vi "RxTx.vi"(8 "error in (no error)":errorcluster) -> (0 "error out":errorcluster)   [LabVIEW 2018]
uses:
  RxTx/RxTx.lvclass
  RxTx/RxTx.lvclass/RxTx.ctl
  <vilib>/addons/_JKI Toolkits/Caraya/classes/Assert/Assert Equal Value_Variant.vi
  <vilib>/addons/_JKI Toolkits/Caraya/classes/Assert/Assert Error.vi
  <vilib>/addons/_JKI Toolkits/Caraya/classes/Test/Test.lvclass
  <vilib>/addons/_JKI Toolkits/Caraya/classes/Assert/Assert.lvclass
panel:
  in  "RxTx in 2":refnum<class "RxTx.lvclass">
  in  "RxTx in":refnum<class "RxTx.lvclass">
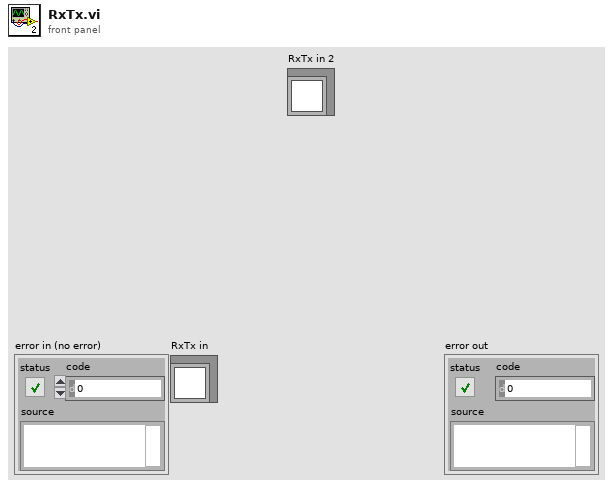
[diagram p1: front panel]
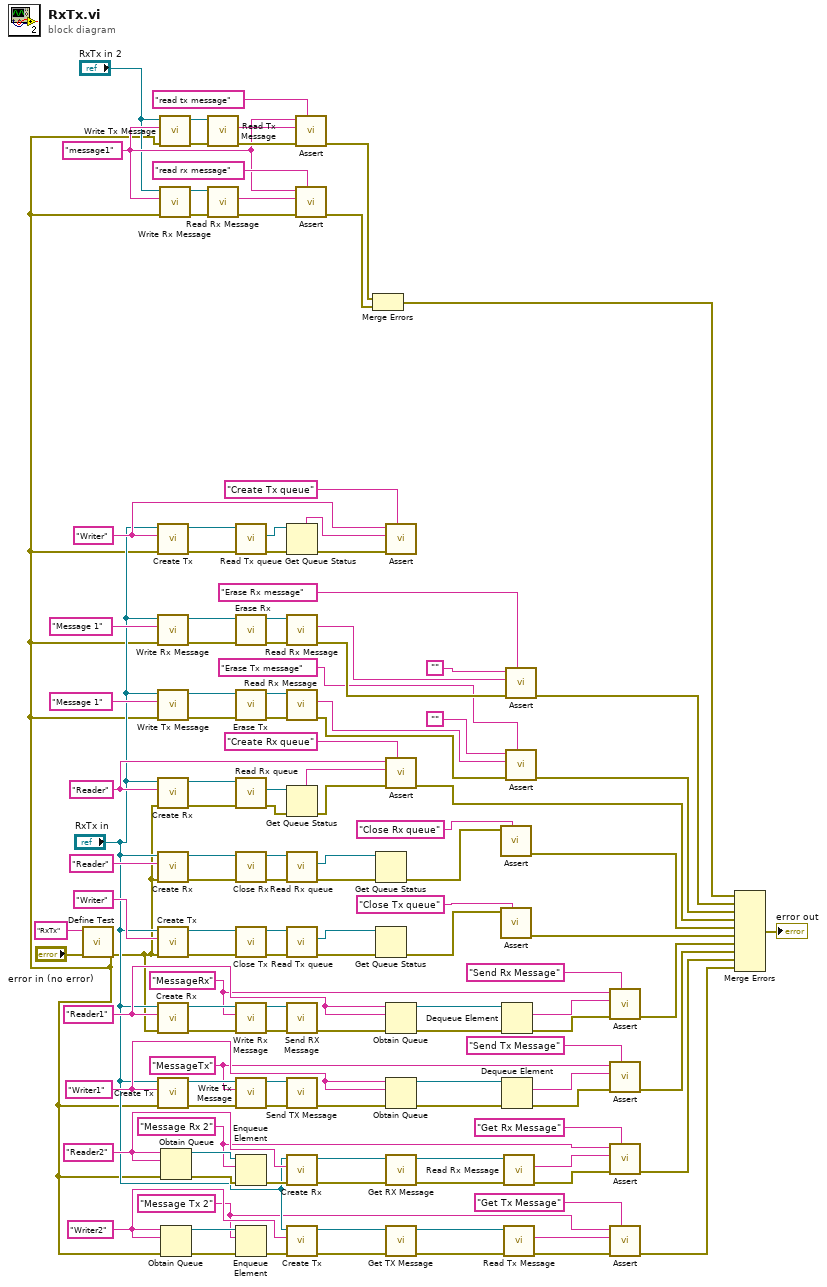
[diagram p0: block diagram]
diagram:
  w4 = "message1" ("Label (VI Title)")
  w18 = "Message Tx 2" ("Rx Message")
  w26 = "Writer2" ("Rx Message")
  w33 = "Message Rx 2" ("Rx Message")
  w40 = "Reader2" ("Rx Message")
  w46 = "MessageTx" ("Rx Message")
  w48 = "Writer1" ("Rx Message")
  w60 = "MessageRx" ("Rx Message")
  w64 = "Reader1" ("Rx Message")
  w97 = "Writer" ("Rx Message")
  w100 = "Reader" ("Rx Message")
  n1 = call <vilib>:"Define Test.vi"("error in (no error)"="error in (no error)", "Label (VI Title)"="RxTx") -> ("error out"=w2:errorcluster)  [unwired: 8 in, 1 out]
  n2 = call "Create Tx.vi"("error in (no error)"=w2, "Writer Name"=w97, "RxTx in"="RxTx in") -> ("error out"=w91:errorcluster, "RxTx out"=w92:refnum<class "RxTx.lvclass">)  [unwired: 7 in]
  n3 = call "Write Rx Message.vi"("error in (no error)"=w2, "Rx Message"="Message 1", "RxTx in"="RxTx in") -> ("error out"=w126:errorcluster, "RxTx out"=w125:refnum<class "RxTx.lvclass">)  [unwired: 7 in]
  n4 = call "Write Tx Message.vi"("error in (no error)"=w2, "Tx Message"="Message 1" ("Rx Message"), "RxTx in"="RxTx in") -> ("error out"=w112:errorcluster, "RxTx out"=w111:refnum<class "RxTx.lvclass">)  [unwired: 7 in]
  n5 = call "Create Rx.vi"("error in (no error)"=w2, "Reader Name"=w100, "RxTx in"="RxTx in") -> ("error out"=w106:errorcluster, "RxTx out"=w105:refnum<class "RxTx.lvclass">)  [unwired: 7 in]
  n6 = call "Create Rx.vi"("error in (no error)"=w2, "Reader Name"="Reader" ("Rx Message"), "RxTx in"="RxTx in") -> ("error out"=w88:errorcluster, "RxTx out"=w87:refnum<class "RxTx.lvclass">)  [unwired: 7 in]
  n7 = call "Create Tx.vi"("error in (no error)"=w2, "Writer Name"="Writer" ("Rx Message"), "RxTx in"="RxTx in") -> ("error out"=w79:errorcluster, "RxTx out"=w78:refnum<class "RxTx.lvclass">)  [unwired: 7 in]
  n8 = call "Create Rx.vi"("error in (no error)"=w2, "Reader Name"=w64, "RxTx in"="RxTx in") -> ("error out"=w69:errorcluster, "RxTx out"=w66:refnum<class "RxTx.lvclass">)  [unwired: 7 in]
  n9 = call "Create Tx.vi"("error in (no error)"=w2, "Writer Name"=w48, "RxTx in"="RxTx in") -> ("error out"=w56:errorcluster, "RxTx out"=w55:refnum<class "RxTx.lvclass">)  [unwired: 7 in]
  n10 = call "Write Tx Message.vi"("error in (no error)"=w2, "Tx Message"=w4, "RxTx in"="RxTx in 2") -> ("error out"=w15:errorcluster, "RxTx out"=w8:refnum<class "RxTx.lvclass">)  [unwired: 7 in]
  n11 = call "Write Rx Message.vi"("error in (no error)"=w2, "Rx Message"=w4, "RxTx in"="RxTx in 2") -> ("error out"=w13:errorcluster, "RxTx out"=w7:refnum<class "RxTx.lvclass">)  [unwired: 7 in]
  n12 = Obtain Queue(name (unnamed)=w40, element data type=w40, error in (no error)=w2) -> (queue out=w42:refnum<queue>, error out=w43:errorcluster)  [unwired: 2 in, 1 out]
  n13 = Obtain Queue(name (unnamed)=w26, element data type=w26, error in (no error)=w2) -> (queue out=w30:refnum<queue>, error out=w29:errorcluster)  [unwired: 2 in, 1 out]
  n14 = call "Read Tx Message.vi"("error in (no error)"=w15, "RxTx in"=w8) -> ("error out"=w14:errorcluster, "Tx Message"=w5:string)  [unwired: 7 in, 1 out]
  n15 = call "Read Rx Message.vi"("error in (no error)"=w13, "RxTx in"=w7) -> ("error out"=w12:errorcluster, "Rx Message"=w6:string)  [unwired: 7 in, 1 out]
  n16 = call "Read Tx queue.vi"("error in (no error)"=w91, "RxTx in"=w92) -> ("error out"=w94:errorcluster, "Tx"=w93:refnum<queue>)  [unwired: 7 in, 1 out]
  n17 = call "Erase Rx.vi"("error in (no error)"=w126, "RxTx in"=w125) -> ("error out"=w124:errorcluster, "RxTx out"=w119:refnum<class "RxTx.lvclass">)  [unwired: 8 in]
  n18 = call "Erase Tx.vi"("error in (no error)"=w112, "RxTx in"=w111) -> ("error out"=w109:errorcluster, "RxTx out"=w110:refnum<class "RxTx.lvclass">)  [unwired: 8 in]
  n19 = call "Read Rx queue.vi"("error in (no error)"=w106, "RxTx in"=w105) -> ("error out"=w103:errorcluster, "Rx"=w104:refnum<queue>)  [unwired: 7 in, 1 out]
  n20 = call "Close Rx.vi"("error in (no error)"=w88, "RxTx in"=w87) -> ("error out"=w86:errorcluster, "RxTx out"=w85:refnum<class "RxTx.lvclass">)  [unwired: 8 in]
  n21 = call "Close Tx.vi"("error in (no error)"=w79, "RxTx in"=w78) -> ("error out"=w76:errorcluster, "RxTx out"=w75:refnum<class "RxTx.lvclass">)  [unwired: 8 in]
  n22 = call "Write Rx Message.vi"("error in (no error)"=w69, "Rx Message"=w60, "RxTx in"=w66) -> ("error out"=w68:errorcluster, "RxTx out"=w67:refnum<class "RxTx.lvclass">)  [unwired: 7 in]
  n23 = call "Write Tx Message.vi"("error in (no error)"=w56, "Tx Message"=w46, "RxTx in"=w55) -> ("error out"=w54:errorcluster, "RxTx out"=w53:refnum<class "RxTx.lvclass">)  [unwired: 7 in]
  n24 = Enqueue Element(queue=w42, element=w33, error in (no error)=w43) -> (error out=w41:errorcluster)  [unwired: 1 in, 2 out]
  n25 = Enqueue Element(queue=w30, element=w18, error in (no error)=w29) -> (error out=w28:errorcluster)  [unwired: 1 in, 2 out]
  n26 = Get Queue Status(queue=w93, error in (no error)=w94) -> (queue name=w96:string, error out=w95:errorcluster)  [unwired: 1 in, 6 out]
  n27 = call "Read Rx Message.vi"("error in (no error)"=w124, "RxTx in"=w119) -> ("error out"=w123:errorcluster, "Rx Message"=w122:string)  [unwired: 7 in, 1 out]
  n28 = call "Read Rx Message.vi"("error in (no error)"=w109, "RxTx in"=w110) -> ("error out"=w113:errorcluster, "Rx Message"=w114:string)  [unwired: 7 in, 1 out]
  n29 = Get Queue Status(queue=w104, error in (no error)=w103) -> (queue name=w101:string, error out=w102:errorcluster)  [unwired: 1 in, 6 out]
  n30 = call "Read Rx queue.vi"("error in (no error)"=w86, "RxTx in"=w85) -> ("error out"=w82:errorcluster, "Rx"=w84:refnum<queue>)  [unwired: 7 in, 1 out]
  n31 = call "Read Tx queue.vi"("error in (no error)"=w76, "RxTx in"=w75) -> ("error out"=w73:errorcluster, "Tx"=w74:refnum<queue>)  [unwired: 7 in, 1 out]
  n32 = call "Send RX Message.vi"("error in (no error)"=w68, "RxTx in"=w67) -> ("error out"=w65:errorcluster)  [unwired: 8 in, 1 out]
  n33 = call "Send TX Message.vi"("error in (no error)"=w54, "RxTx in"=w53) -> ("error out"=w52:errorcluster)  [unwired: 8 in, 1 out]
  n34 = call "Create Rx.vi"("error in (no error)"=w41, "Reader Name"=w40, "RxTx in"="RxTx in") -> ("error out"=w39:errorcluster, "RxTx out"=w38:refnum<class "RxTx.lvclass">)  [unwired: 7 in]
  n35 = call "Create Tx.vi"("error in (no error)"=w28, "Writer Name"=w26, "RxTx in"="RxTx in") -> ("error out"=w24:errorcluster, "RxTx out"=w25:refnum<class "RxTx.lvclass">)  [unwired: 7 in]
  n36 = call-poly <vilib>:"Assert.vi"("Label"="read tx message" ("Label (VI Title)"), "error in (no error)"=w14, "Actual"=w5, "Expected"=w4) -> ("error out"=w16:errorcluster)  [unwired: 6 in, 1 out]
  n37 = call-poly <vilib>:"Assert.vi"("Label"="read rx message" ("Label (VI Title)"), "error in (no error)"=w12, "Actual"=w6, "Expected"=w4) -> ("error out"=w11:errorcluster)  [unwired: 6 in, 1 out]
  n38 = Merge Errors(w16, w11) -> (w1:errorcluster)
  n39 = Get Queue Status(queue=w84, error in (no error)=w82) -> (error out=w83:errorcluster)  [unwired: 1 in, 7 out]
  n40 = Get Queue Status(queue=w74, error in (no error)=w73) -> (error out=w72:errorcluster)  [unwired: 1 in, 7 out]
  n41 = call-poly <vilib>:"Assert.vi"("Label"="Create Tx queue" ("Label (VI Title)"), "error in (no error)"=w95, "Actual"=w96, "Expected"=w97) -> ()  [unwired: 6 in, 2 out]
  n42 = call-poly <vilib>:"Assert.vi"("Label"="Create Rx queue" ("Label (VI Title)"), "error in (no error)"=w102, "Actual"=w101, "Expected"=w100) -> ("error out"=w99:errorcluster)  [unwired: 6 in, 1 out]
  n43 = Obtain Queue(name (unnamed)=w64, element data type=w64, error in (no error)=w65) -> (queue out=w63:refnum<queue>, error out=w62:errorcluster)  [unwired: 2 in, 1 out]
  n44 = Obtain Queue(name (unnamed)=w48, element data type=w48, error in (no error)=w52) -> (queue out=w49:refnum<queue>, error out=w51:errorcluster)  [unwired: 2 in, 1 out]
  n45 = call "Get RX Message.vi"("error in (no error)"=w39, "RxTx in"=w38) -> ("error out"=w37:errorcluster, "RxTx out"=w36:refnum<class "RxTx.lvclass">)  [unwired: 8 in]
  n46 = call "Get TX Message.vi"("error in (no error)"=w24, "RxTx in"=w25) -> ("error out"=w23:errorcluster, "RxTx out"=w22:refnum<class "RxTx.lvclass">)  [unwired: 8 in]
  n47 = call-poly <vilib>:"Assert.vi"("Label"="Close Rx queue" ("Label (VI Title)"), "Error?"=w83) -> ("error out"=w81:errorcluster)  [unwired: 8 in, 1 out]
  n48 = call-poly <vilib>:"Assert.vi"("Label"="Close Tx queue" ("Label (VI Title)"), "Error?"=w72) -> ("error out"=w71:errorcluster)  [unwired: 8 in, 1 out]
  n49 = Dequeue Element(queue=w63, error in (no error)=w62) -> (element=w61:string, error out=w59:errorcluster)  [unwired: 1 in, 2 out]
  n50 = Dequeue Element(queue=w49, error in (no error)=w51) -> (element=w47:string, error out=w50:errorcluster)  [unwired: 1 in, 2 out]
  n51 = call "Read Rx Message.vi"("error in (no error)"=w37, "RxTx in"=w36) -> ("error out"=w35:errorcluster, "Rx Message"=w34:string)  [unwired: 7 in, 1 out]
  n52 = call "Read Tx Message.vi"("error in (no error)"=w23, "RxTx in"=w22) -> ("error out"=w21:errorcluster, "Tx Message"=w19:string)  [unwired: 7 in, 1 out]
  n53 = call-poly <vilib>:"Assert.vi"("Label"="Erase Rx message" ("Label (VI Title)"), "error in (no error)"=w123, "Actual"=w122, "Expected"="") -> ("error out"=w118:errorcluster)  [unwired: 6 in, 1 out]
  n54 = call-poly <vilib>:"Assert.vi"("Label"="Erase Tx message" ("Label (VI Title)"), "error in (no error)"=w113, "Actual"=w114, "Expected"="") -> ("error out"=w108:errorcluster)  [unwired: 6 in, 1 out]
  n55 = call-poly <vilib>:"Assert.vi"("Label"="Send Rx Message" ("Label (VI Title)"), "error in (no error)"=w59, "Actual"=w61, "Expected"=w60) -> ("error out"=w58:errorcluster)  [unwired: 6 in, 1 out]
  n56 = call-poly <vilib>:"Assert.vi"("Label"="Send Tx Message" ("Label (VI Title)"), "error in (no error)"=w50, "Actual"=w47, "Expected"=w46) -> ("error out"=w44:errorcluster)  [unwired: 6 in, 1 out]
  n57 = call-poly <vilib>:"Assert.vi"("Label"="Get Rx Message" ("Label (VI Title)"), "error in (no error)"=w35, "Actual"=w34, "Expected"=w33) -> ("error out"=w32:errorcluster)  [unwired: 6 in, 1 out]
  n58 = call-poly <vilib>:"Assert.vi"("Label"="Get Tx Message" ("Label (VI Title)"), "error in (no error)"=w21, "Actual"=w19, "Expected"=w18) -> ("error out"=w20:errorcluster)  [unwired: 6 in, 1 out]
  n59 = Merge Errors(w1, w118, w108, w99, w81, w71, w58, w44, w32, w20) -> (→"error out":errorcluster)
